vi "#129_MAV_MSG_SCALED_IMU3_DECODE.vi"(11 "mavlink_payload":u8[](array[numeric])) -> (3 "SCALED_IMU3":T1)   [LabVIEW 2023]
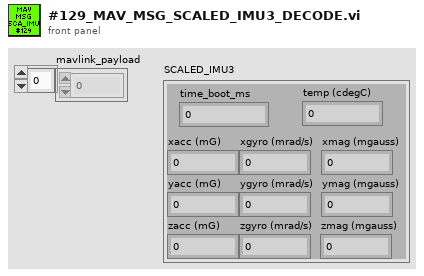
[diagram p1: front panel]
types:
  T1 = cluster{"time_boot_ms":u32, "xacc (mG)":i16, "yacc (mG)":i16, "zacc (mG)":i16, "xgyro (mrad/s)":i16, "ygyro (mrad/s)":i16, "zgyro (mrad/s)":i16, "xmag (mgauss)":i16, "ymag (mgauss)":i16, "zmag (mgauss)":i16, "temp (cdegC)":i16}
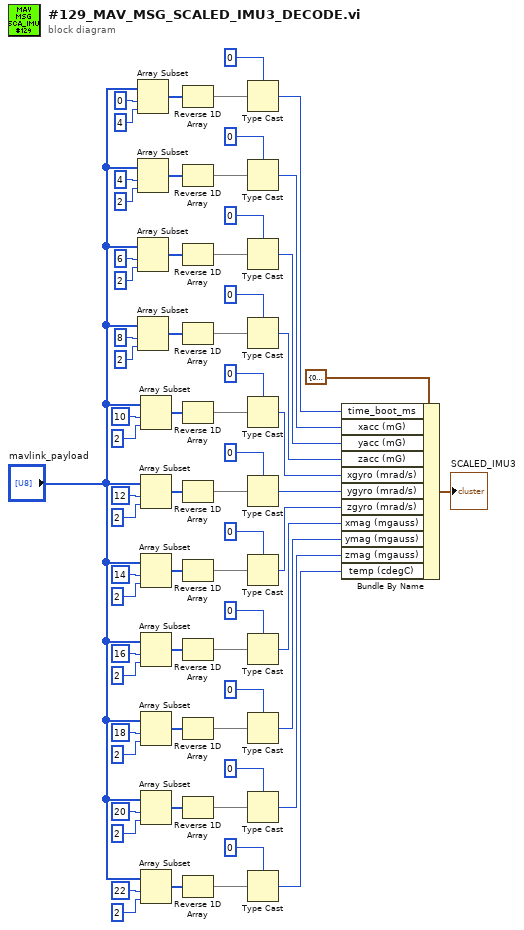
[diagram p0: block diagram]
diagram:
  n1 = Array Subset(array="mavlink_payload", index=0 ("Index"), length=4) -> (w68:u8[])
  n2 = Array Subset(array="mavlink_payload", index=4 ("Index"), length=2) -> (w63:u8[])
  n3 = Array Subset(array="mavlink_payload", index=6 ("Index"), length=2) -> (w58:u8[])
  n4 = Array Subset(array="mavlink_payload", index=8 ("Index"), length=2) -> (w53:u8[])
  n5 = Array Subset(array="mavlink_payload", index=10 ("Index"), length=2) -> (w48:u8[])
  n6 = Array Subset(array="mavlink_payload", index=12 ("Index"), length=2) -> (w43:u8[])
  n7 = Array Subset(array="mavlink_payload", index=14 ("Index"), length=2) -> (w38:u8[])
  n8 = Array Subset(array="mavlink_payload", index=16 ("Index"), length=2) -> (w33:u8[])
  n9 = Array Subset(array="mavlink_payload", index=18 ("Index"), length=2) -> (w28:u8[])
  n10 = Array Subset(array="mavlink_payload", index=20 ("Index"), length=2) -> (w23:u8[])
  n11 = Array Subset(array="mavlink_payload", index=22 ("Index"), length=2) -> (w18:u8[])
  n12 = Reverse 1D Array(array=w68) -> (reversed array=w67:u8[])
  n13 = Reverse 1D Array(array=w63) -> (reversed array=w62:u8[])
  n14 = Reverse 1D Array(array=w58) -> (reversed array=w57:u8[])
  n15 = Reverse 1D Array(array=w53) -> (reversed array=w52:u8[])
  n16 = Reverse 1D Array(array=w48) -> (reversed array=w47:u8[])
  n17 = Reverse 1D Array(array=w43) -> (reversed array=w42:u8[])
  n18 = Reverse 1D Array(array=w38) -> (reversed array=w37:u8[])
  n19 = Reverse 1D Array(array=w33) -> (reversed array=w32:u8[])
  n20 = Reverse 1D Array(array=w28) -> (reversed array=w27:u8[])
  n21 = Reverse 1D Array(array=w23) -> (reversed array=w22:u8[])
  n22 = Reverse 1D Array(array=w18) -> (reversed array=w17:u8[])
  n23 = Type Cast(type=u32 0 ("Index"), x=w67) -> (*(type *) &x=w11:u32)
  n24 = Type Cast(type=i16 0 ("Index"), x=w62) -> (*(type *) &x=w10:i16)
  n25 = Type Cast(type=i16 0 ("Index"), x=w57) -> (*(type *) &x=w9:i16)
  n26 = Type Cast(type=i16 0 ("Index"), x=w52) -> (*(type *) &x=w8:i16)
  n27 = Type Cast(type=i16 0 ("Index"), x=w47) -> (*(type *) &x=w7:i16)
  n28 = Type Cast(type=i16 0 ("Index"), x=w42) -> (*(type *) &x=w6:i16)
  n29 = Type Cast(type=i16 0 ("Index"), x=w37) -> (*(type *) &x=w5:i16)
  n30 = Type Cast(type=i16 0 ("Index"), x=w32) -> (*(type *) &x=w4:i16)
  n31 = Type Cast(type=i16 0 ("Index"), x=w27) -> (*(type *) &x=w3:i16)
  n32 = Type Cast(type=i16 0 ("Index"), x=w22) -> (*(type *) &x=w2:i16)
  n33 = Type Cast(type=i16 0 ("Index"), x=w17) -> (*(type *) &x=w1:i16)
  n34 = Bundle By Name(cluster=T1 {"time_boot_ms"=0, "xacc (mG)"=0, "yacc (mG)"=0, "zacc (mG)"=0, "xgyro (mrad/s)"=0, "ygyro (mrad/s)"=0, "zgyro (mrad/s)"=0, "xmag (mgauss)"=0, "ymag (mgauss)"=0, "zmag (mgauss)"=0, "temp (cdegC)"=0} ("SCALED_IMU3"), "time_boot_ms"=w11, "xacc (mG)"=w10, "yacc (mG)"=w9, "zacc (mG)"=w8, "xgyro (mrad/s)"=w7, "ygyro (mrad/s)"=w6, "zgyro (mrad/s)"=w5, "xmag (mgauss)"=w4, "ymag (mgauss)"=w3, "zmag (mgauss)"=w2, "temp (cdegC)"=w1) -> (→"SCALED_IMU3":T1)
